vi "Update Graphs.vi"(8 "error in (no error)":errorcluster, 11 "OD600 in":refnum<class "OD600.lvclass">) -> (0 "error out":errorcluster, 3 "OD600 out":refnum<class "OD600.lvclass">)   [LabVIEW 2013, in "OD600.lvlib" / "OD600.lvclass"]
uses:
  OD600.lvclass
  <vilib>/Analysis/6fits.llb/Curve Fitting Criteria.ctl
  <vilib>/Analysis/NI_AALPro.lvlib
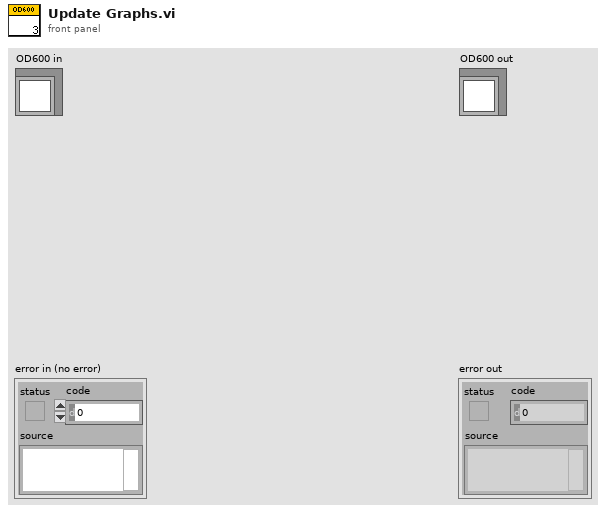
[diagram p1: front panel]
types:
  T1 = cluster{"output array":dbl[], "output array":dbl[]}
  T2 = typedef "NI_AALPro.lvlib/Curve Fitting Criteria.ctl" = u16
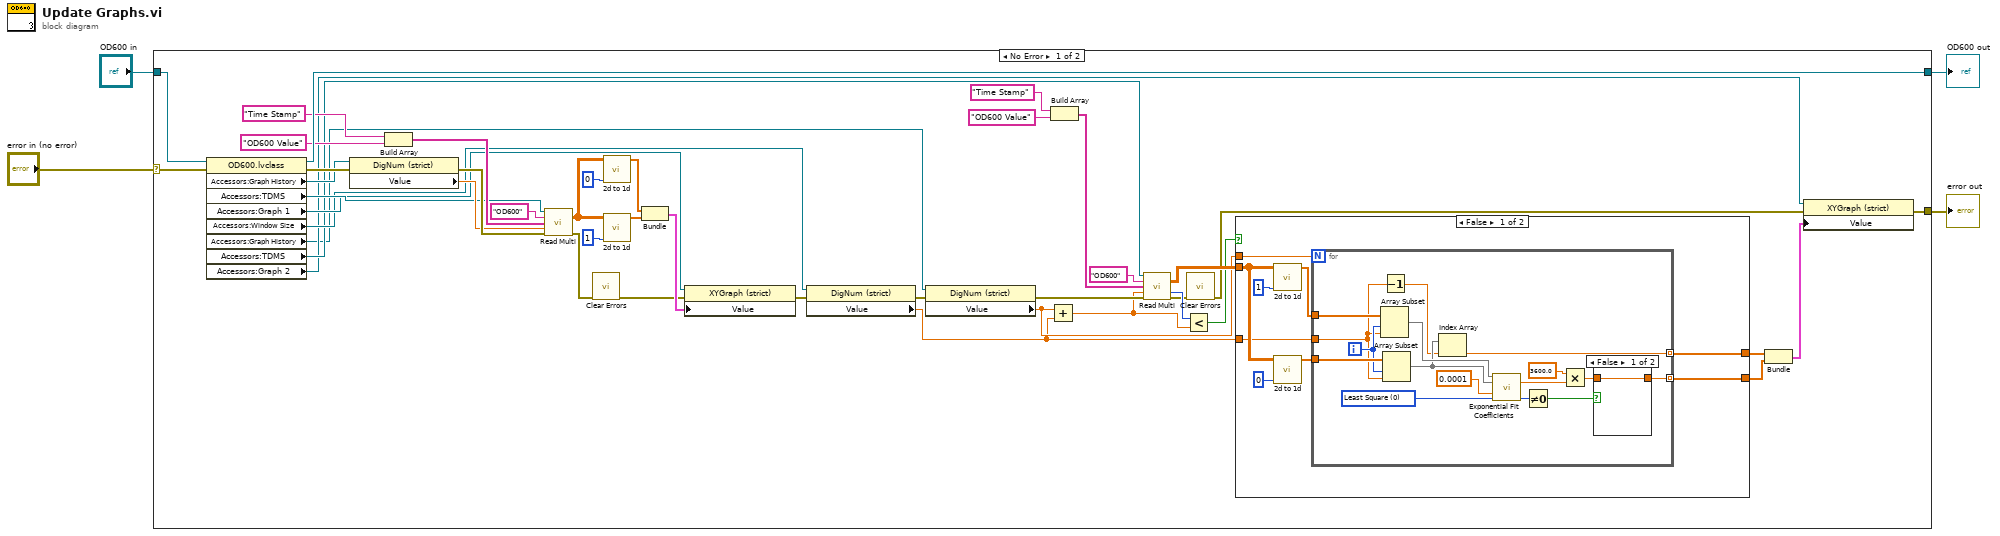
[diagram p0: block diagram]
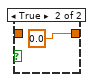
[diagram p2: hidden frame]
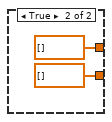
[diagram p3: hidden frame]
diagram:
  n1 = case shown="No Error" "error in (no error)" {
    selector: "error in (no error)" -> [w44 w79]
    tunnel: [w30 w79] -> w2
    tunnel: [w47 w78] -> w1
    tunnel: "OD600 in" -> [w48 w78]
    frame No Error {
      n2 = property class="OD600.lvclass"(reference=w48, error in=w44) -> (reference out=w47:refnum<class "OD600.lvclass">, error out=w43:errorcluster, "Accessors:Graph History"=w37:refnum<vi>, "Accessors:TDMS"=w38:refnum<k34>, "Accessors:Graph 1"=w36:refnum<vi>, "Accessors:Window Size"=w28:refnum<vi>, "Accessors:Graph History"=w17:refnum<vi>, "Accessors:TDMS"=w21:refnum<k34>, "Accessors:Graph 2"=w18:refnum<vi>)
      n3 = property class="DigNum (strict)"(reference=w37, error in=w43) -> (error out=w42:errorcluster, "Value"=w39:dbl)  [unwired: 1 out]
      n4 = Build Array("Time Stamp" ("Channel"), "OD600 Value" ("string")) -> (w40:string[])
      n5 = call "Read Multi.vi"("tdms file in"=w38, "group"="OD600", "Channel"=w40, "Numeric"=w39, "error in (no error)"=w42) -> ("Array"=w31:dbl[][], "error out"=w6:errorcluster)  [unwired: 7 in, 2 out]
      n6 = call <vilib>:"Clear Errors.vi"("error in (no error)"=w6) -> ("error out"=w5:errorcluster)  [unwired: 6 in]
      n7 = call "2d to 1d.vi"("index"=0, "array"=w31) -> ("output array"=w32:dbl[])  [unwired: 9 in]
      n8 = call "2d to 1d.vi"("index"=1, "array"=w31) -> ("output array"=w33:dbl[])  [unwired: 9 in]
      n9 = Bundle("output array"=w32, "output array"=w33) -> (w29:T1)  [unwired: 1 in]
      n10 = property class="XYGraph (strict)"(reference=w36, error in=w5, "Value"=w29) -> (error out=w19:errorcluster)  [unwired: 1 out]
      n11 = property class="DigNum (strict)"(reference=w28, error in=w19) -> (error out=w20:errorcluster, "Value"=w15:dbl)  [unwired: 1 out]
      n12 = property class="DigNum (strict)"(reference=w17, error in=w20) -> (error out=w24:errorcluster, "Value"=w16:dbl)  [unwired: 1 out]
      n13 = Add(x=w16, y=w15) -> (x+y=w10:dbl)
      n14 = Build Array("Time Stamp" ("Channel"), "OD600 Value" ("string")) -> (w26:string[])
      n15 = call "Read Multi.vi"("tdms file in"=w21, "group"="OD600", "Channel"=w26, "Numeric"=w10, "error in (no error)"=w24) -> ("Array"=w27:dbl[][], "Length"=w11:u64, "error out"=w8:errorcluster)  [unwired: 7 in, 1 out]
      n16 = Less?(x=w11, y=w10) -> (x < y?=w9:bool)
      n17 = call <vilib>:"Clear Errors.vi"("error in (no error)"=w8) -> ("error out"=w7:errorcluster)  [unwired: 6 in]
      n18 = case shown="False" w9 {
        tunnel: w27 -> [w57 _]
        tunnel: w16 -> [w53 _]
        tunnel: w15 -> [w52 _]
        tunnel: [w51 dbl[] []] -> w14
        tunnel: [w50 dbl[] []] -> w13
        frame False {
          n19 = call "2d to 1d.vi"("index"=1, "array"=w57) -> ("output array"=w49:dbl[])  [unwired: 9 in]
          n20 = call "2d to 1d.vi"("index"=0, "array"=w57) -> ("output array"=w54:dbl[])  [unwired: 9 in]
          n21 = for {
            N: w53 -> [_]
            tunnel: [w61] -> w50 mode=indexing
            tunnel: w54 -> [w71]
            tunnel: w49 -> [w69]
            tunnel: w52 -> [w66]
            tunnel: [w64] -> w51 mode=indexing
            i -> [w70]
            w73 = T2 0 items=["Least Square", "Least Absolute Residual", "Bisquare"] ("method")
            n22 = Array Subset(array=w69, index=w70, length=w66) -> (w68:dbl[])
            n23 = Decrement(x=w66) -> (x-1=w65:dbl)
            n24 = Array Subset(array=w71, index=w70, length=w66) -> (w67:dbl[])
            n25 = Index Array(array=w67, index=w65) -> (element=w64:dbl)
            n26 = call <vilib>:"Exponential Fit Coefficients.vi"("Y"=w68, "X"=w67, "tolerance"=0.0001, "method"=w73) -> ("damping"=w60:dbl, "error"=w63:i32)  [unwired: 9 in, 1 out]
            n27 = Not Equal To 0?(x=w63) -> (x != 0?=w62:bool)
            n28 = Multiply(x=3600.0, y=w60) -> (x*y=w59:dbl)
            n29 = case shown="False" w62 {
              tunnel: [w74 0.0 ("damping")] -> w61
              tunnel: w59 -> [w74 _]
              frame False {
              }
              frame True {
              }
            }
          }
        }
        frame True {
        }
      }
      n30 = Bundle(w14, w13) -> (w12:cluster{dbl[], dbl[]})  [unwired: 1 in]
      n31 = property class="XYGraph (strict)"(reference=w18, error in=w7, "Value"=w12) -> (error out=w30:errorcluster)  [unwired: 1 out]
    }
    frame Error {
    }
  }
  "error out" <- w2
  "OD600 out" <- w1
